vi "WriteIni.vi"(1 "configuration file path":path=path "E:/LabVIEW/福尔达/AppData") -> ()   [LabVIEW 2018]
uses:
  <vilib>/Utility/config.llb/Write Key (Double).vi
  <vilib>/Utility/config.llb/NI_LVConfig.lvlib
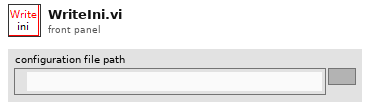
[diagram p1: front panel]
types:
  T1 = typedef "NI_LVConfig.lvlib/Config Data RefNum.ctl" = refnum<k1>
  T2 = cluster{"轮盘预压力":sgl, "泄漏量上限":sgl, "压力上限":sgl, "压力下限":sgl, "风门闭电压上限":sgl, "风门闭电压下限":sgl, "风门开电压上限":sgl, "风门开电压下限":sgl, "LED电流上限":sgl, "LED电流下限":sgl, "气压稳定时间":sgl, "伺服速度":sgl}
  T3 = cluster{"选择":enum16{"Fx", "Fy", "Fz", "Mx", "My", "Mz"}, "系数":sgl, "上限":sgl, "下限":sgl, "Ymax":dbl, "Ymin":dbl, "点数":dbl, "锁系数x":sgl, "锁上限":sgl, "锁下限":sgl, "锁系数+":sgl, "起点":dbl, "终点":dbl, "锁起点":dbl, "锁终点":dbl}
  T4 = cluster{"选择":enum16{"Fx", "Fy", "Fz", "Mx", "My", "Mz"}, "系数":sgl, "上限":sgl, "下限":sgl, "Ymax":dbl, "Ymin":dbl, "点数":dbl, "起点":dbl, "终点":dbl}
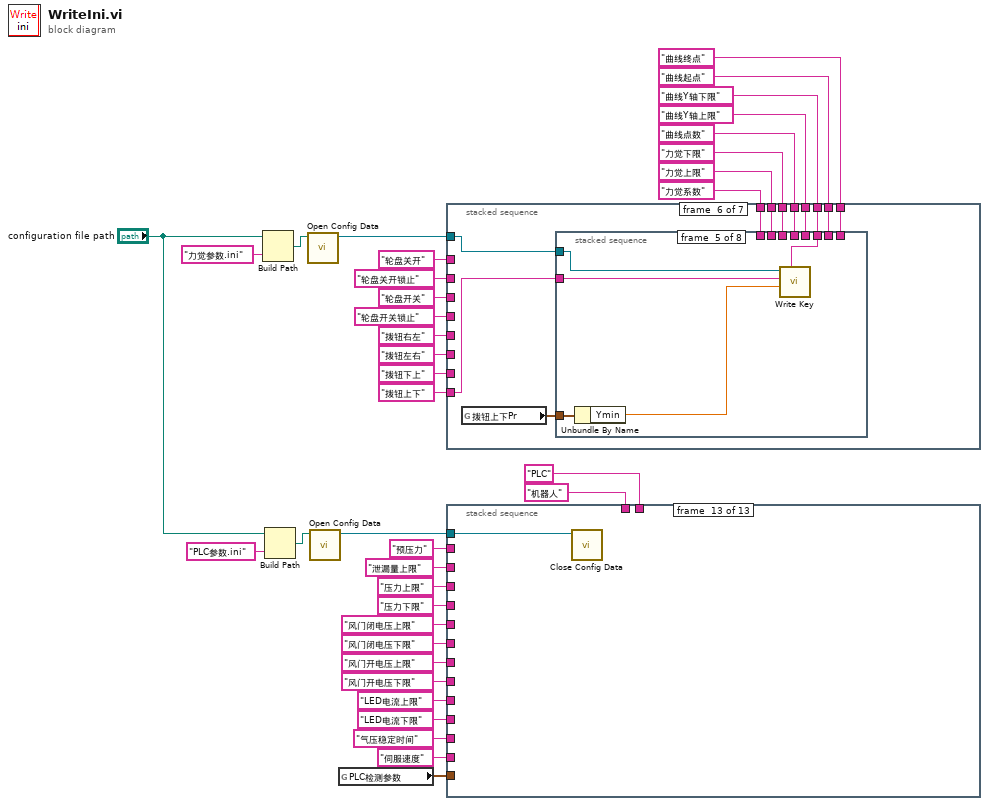
[diagram p0: block diagram]
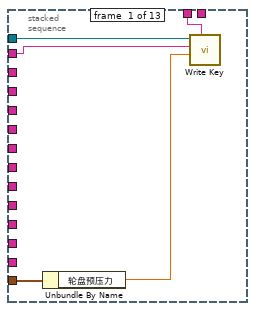
[diagram p2: hidden frame]
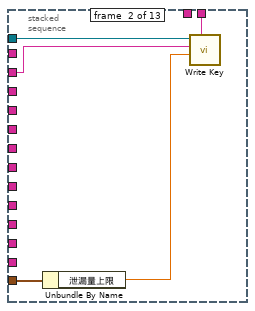
[diagram p3: hidden frame]
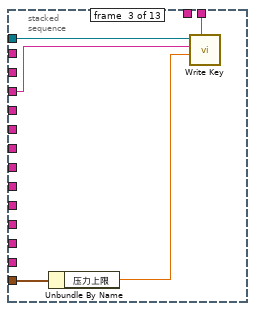
[diagram p4: hidden frame]
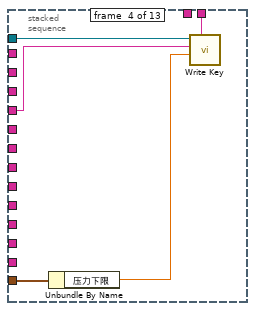
[diagram p5: hidden frame]
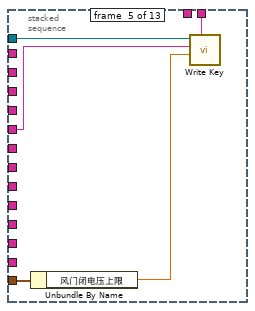
[diagram p6: hidden frame]
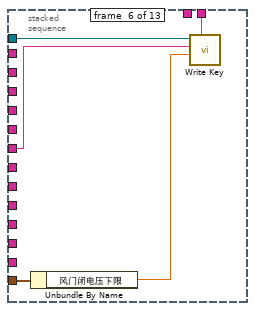
[diagram p7: hidden frame]
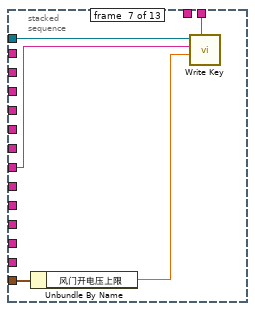
[diagram p8: hidden frame]
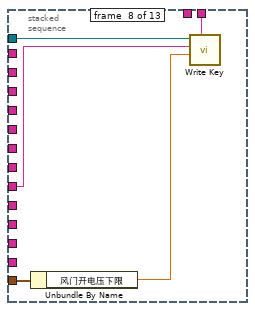
[diagram p9: hidden frame]
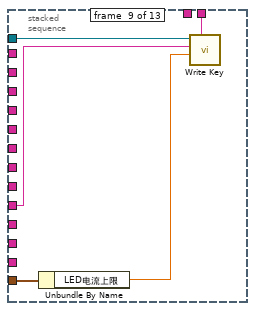
[diagram p10: hidden frame]
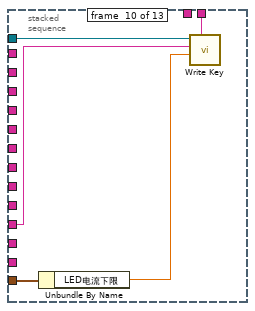
[diagram p11: hidden frame]
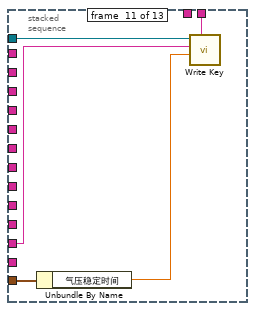
[diagram p12: hidden frame]
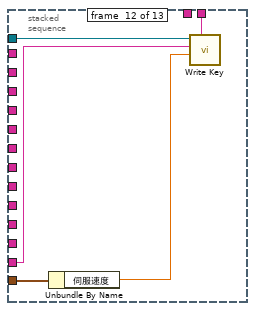
[diagram p13: hidden frame]
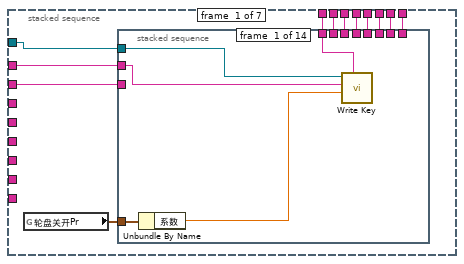
[diagram p14: hidden frame]
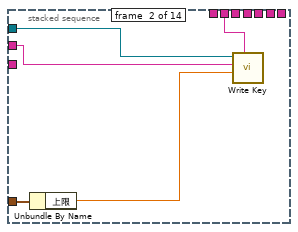
[diagram p15: hidden frame]
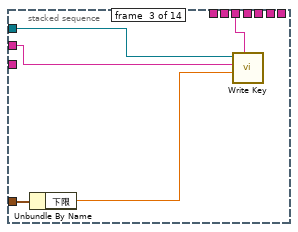
[diagram p16: hidden frame]
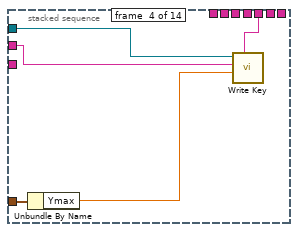
[diagram p17: hidden frame]
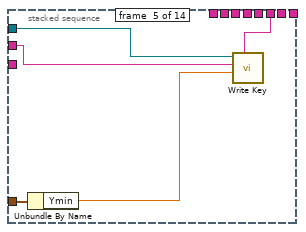
[diagram p18: hidden frame]
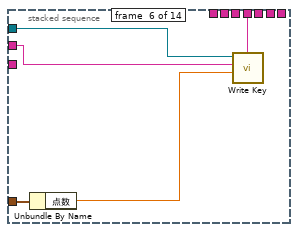
[diagram p19: hidden frame]
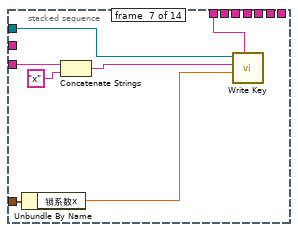
[diagram p20: hidden frame]
diagram:
  n1 = Build Path(base path="configuration file path", name or relative path="力觉参数.ini" ("名称或相对路径")) -> (appended path=w22:path)
  n2 = Build Path(base path="configuration file path", name or relative path="PLC参数.ini" ("名称或相对路径")) -> (appended path=w18:path)
  n3 = call <vilib>:"Open Config Data.vi"("configuration file path"=w22) -> ("refnum"=w20:T1)  [unwired: 8 in, 2 out]
  n4 = call <vilib>:"Open Config Data.vi"("configuration file path"=w18) -> ("refnum"=w17:T1)  [unwired: 8 in, 2 out]
  n5 = global read "全局 1.vi" "PLC检测参数"() -> (w19:T2)
  n6 = stacked-sequence {
    tunnel: w20 -> [w39 w125 w211 w262 w313 w364 w415]
    tunnel: "轮盘关开" -> [w49 _ _ _ _ _ _]
    tunnel: "拨钮上下" -> [_ _ _ _ _ w365 _]
    tunnel: "拨钮下上" -> [_ _ _ _ w314 _ _]
    tunnel: "拨钮左右" -> [_ _ _ w263 _ _ _]
    tunnel: "拨钮右左" -> [_ _ w212 _ _ _ _]
    tunnel: "轮盘开关锁止" -> [_ w126 _ _ _ _ _]
    tunnel: "轮盘开关" -> [_ w127 _ _ _ _ _]
    tunnel: "轮盘关开锁止" -> [w40 _ _ _ _ _ _]
    tunnel: "力觉系数" -> [w48 w135 w220 w271 w322 w373 _]
    tunnel: "力觉上限" -> [w47 w134 w219 w270 w321 w372 _]
    tunnel: "力觉下限" -> [w46 w133 w218 w269 w320 w371 _]
    tunnel: "曲线点数" -> [w45 w132 w217 w268 w319 w370 _]
    tunnel: "曲线Y轴上限" -> [w44 w131 w216 w267 w318 w369 _]
    tunnel: "曲线Y轴下限" -> [w43 w130 w215 w266 w317 w368 _]
    tunnel: "曲线起点" -> [w42 w129 w214 w265 w316 w367 _]
    tunnel: "曲线终点" -> [w41 w128 w213 w264 w315 w366 _]
    frame #0 {
      n7 = global read "全局 1.vi" "轮盘关开Pr"() -> (w50:T3)
      n8 = stacked-sequence {
        tunnel: w49 -> [w52 w57 w62 w67 w72 w77 _ _ _ _ w106 w111 _ _]
        tunnel: w50 -> [w55 w60 w65 w70 w75 w80 w87 w92 w97 w104 w109 w114 w119 w124]
        tunnel: w39 -> [w53 w58 w63 w68 w73 w78 w85 w90 w95 w102 w107 w112 w117 w122]
        tunnel: w48 -> [w51 _ _ _ _ _ w84 _ _ w98 _ _ _ _]
        tunnel: w47 -> [_ w56 _ _ _ _ _ w88 _ _ _ _ _ _]
        tunnel: w46 -> [_ _ w61 _ _ _ _ _ w93 _ _ _ _ _]
        tunnel: w45 -> [_ _ _ _ _ w76 _ _ _ _ _ _ _ _]
        tunnel: w44 -> [_ _ _ w66 _ _ _ _ _ _ _ _ _ _]
        tunnel: w43 -> [_ _ _ _ w71 _ _ _ _ _ _ _ _ _]
        tunnel: w42 -> [_ _ _ _ _ _ _ _ _ _ w105 _ w115 _]
        tunnel: w41 -> [_ _ _ _ _ _ _ _ _ _ _ w110 _ w120]
        tunnel: w40 -> [_ _ _ _ _ _ w83 w89 w94 w101 _ _ w116 w121]
        frame #0 {
          n9 = Unbundle By Name(w55) -> ("系数"=w54:sgl)
          n10 = call-poly <vilib>:"Write Key.vi"("section"=w51, "value"=w54, "key"=w52, "refnum"=w53) -> ()  [unwired: 5 in, 3 out]
        }
        frame #1 {
          n11 = Unbundle By Name(w60) -> ("上限"=w59:sgl)
          n12 = call-poly <vilib>:"Write Key.vi"("section"=w56, "value"=w59, "key"=w57, "refnum"=w58) -> ()  [unwired: 5 in, 3 out]
        }
        frame #2 {
          n13 = Unbundle By Name(w65) -> ("下限"=w64:sgl)
          n14 = call-poly <vilib>:"Write Key.vi"("section"=w61, "value"=w64, "key"=w62, "refnum"=w63) -> ()  [unwired: 5 in, 3 out]
        }
        frame #3 {
          n15 = Unbundle By Name(w70) -> ("Ymax"=w69:dbl)
          n16 = call-poly <vilib>:"Write Key.vi"("section"=w66, "value"=w69, "key"=w67, "refnum"=w68) -> ()  [unwired: 5 in, 3 out]
        }
        frame #4 {
          n17 = Unbundle By Name(w75) -> ("Ymin"=w74:dbl)
          n18 = call-poly <vilib>:"Write Key.vi"("section"=w71, "value"=w74, "key"=w72, "refnum"=w73) -> ()  [unwired: 5 in, 3 out]
        }
        frame #5 {
          n19 = Unbundle By Name(w80) -> ("点数"=w79:dbl)
          n20 = call-poly <vilib>:"Write Key.vi"("section"=w76, "value"=w79, "key"=w77, "refnum"=w78) -> ()  [unwired: 5 in, 3 out]
        }
        frame #6 {
          n21 = Unbundle By Name(w87) -> ("锁系数x"=w86:sgl)
          n22 = Concatenate Strings(w83, "x") -> (w82:string)
          n23 = call-poly <vilib>:"Write Key.vi"("section"=w84, "value"=w86, "key"=w82, "refnum"=w85) -> ()  [unwired: 5 in, 3 out]
        }
        frame #7 {
          n24 = Unbundle By Name(w92) -> ("锁上限"=w91:sgl)
          n25 = call-poly <vilib>:"Write Key.vi"("section"=w88, "value"=w91, "key"=w89, "refnum"=w90) -> ()  [unwired: 5 in, 3 out]
        }
        frame #8 {
          n26 = Unbundle By Name(w97) -> ("锁下限"=w96:sgl)
          n27 = call-poly <vilib>:"Write Key.vi"("section"=w93, "value"=w96, "key"=w94, "refnum"=w95) -> ()  [unwired: 5 in, 3 out]
        }
        frame #9 {
          n28 = Unbundle By Name(w104) -> ("锁系数+"=w103:sgl)
          n29 = Concatenate Strings(w101, "+") -> (w100:string)
          n30 = call-poly <vilib>:"Write Key.vi"("section"=w98, "value"=w103, "key"=w100, "refnum"=w102) -> ()  [unwired: 5 in, 3 out]
        }
        frame #10 {
          n31 = Unbundle By Name(w109) -> ("起点"=w108:dbl)
          n32 = call-poly <vilib>:"Write Key.vi"("section"=w105, "value"=w108, "key"=w106, "refnum"=w107) -> ()  [unwired: 5 in, 3 out]
        }
        frame #11 {
          n33 = Unbundle By Name(w114) -> ("终点"=w113:dbl)
          n34 = call-poly <vilib>:"Write Key.vi"("section"=w110, "value"=w113, "key"=w111, "refnum"=w112) -> ()  [unwired: 5 in, 3 out]
        }
        frame #12 {
          n35 = Unbundle By Name(w119) -> ("锁起点"=w118:dbl)
          n36 = call-poly <vilib>:"Write Key.vi"("section"=w115, "value"=w118, "key"=w116, "refnum"=w117) -> ()  [unwired: 5 in, 3 out]
        }
        frame #13 {
          n37 = Unbundle By Name(w124) -> ("锁终点"=w123:dbl)
          n38 = call-poly <vilib>:"Write Key.vi"("section"=w120, "value"=w123, "key"=w121, "refnum"=w122) -> ()  [unwired: 5 in, 3 out]
        }
      }
    }
    frame #1 {
      n39 = global read "全局 1.vi" "轮盘开关Pr"() -> (w136:T3)
      n40 = stacked-sequence {
        tunnel: w127 -> [w138 w143 w148 w153 w158 w163 _ _ _ _ w192 w197 _ _]
        tunnel: w136 -> [w141 w146 w151 w156 w161 w166 w173 w178 w183 w190 w195 w200 w205 w210]
        tunnel: w125 -> [w139 w144 w149 w154 w159 w164 w171 w176 w181 w188 w193 w198 w203 w208]
        tunnel: w135 -> [w137 _ _ _ _ _ w170 _ _ w184 _ _ _ _]
        tunnel: w134 -> [_ w142 _ _ _ _ _ w174 _ _ _ _ _ _]
        tunnel: w133 -> [_ _ w147 _ _ _ _ _ w179 _ _ _ _ _]
        tunnel: w132 -> [_ _ _ _ _ w162 _ _ _ _ _ _ _ _]
        tunnel: w131 -> [_ _ _ w152 _ _ _ _ _ _ _ _ _ _]
        tunnel: w130 -> [_ _ _ _ w157 _ _ _ _ _ _ _ _ _]
        tunnel: w129 -> [_ _ _ _ _ _ _ _ _ _ w191 _ w201 _]
        tunnel: w128 -> [_ _ _ _ _ _ _ _ _ _ _ w196 _ w206]
        tunnel: w126 -> [_ _ _ _ _ _ w169 w175 w180 w187 _ _ w202 w207]
        frame #0 {
          n41 = Unbundle By Name(w141) -> ("系数"=w140:sgl)
          n42 = call-poly <vilib>:"Write Key.vi"("section"=w137, "value"=w140, "key"=w138, "refnum"=w139) -> ()  [unwired: 5 in, 3 out]
        }
        frame #1 {
          n43 = Unbundle By Name(w146) -> ("上限"=w145:sgl)
          n44 = call-poly <vilib>:"Write Key.vi"("section"=w142, "value"=w145, "key"=w143, "refnum"=w144) -> ()  [unwired: 5 in, 3 out]
        }
        frame #2 {
          n45 = Unbundle By Name(w151) -> ("下限"=w150:sgl)
          n46 = call-poly <vilib>:"Write Key.vi"("section"=w147, "value"=w150, "key"=w148, "refnum"=w149) -> ()  [unwired: 5 in, 3 out]
        }
        frame #3 {
          n47 = Unbundle By Name(w156) -> ("Ymax"=w155:dbl)
          n48 = call-poly <vilib>:"Write Key.vi"("section"=w152, "value"=w155, "key"=w153, "refnum"=w154) -> ()  [unwired: 5 in, 3 out]
        }
        frame #4 {
          n49 = Unbundle By Name(w161) -> ("Ymin"=w160:dbl)
          n50 = call-poly <vilib>:"Write Key.vi"("section"=w157, "value"=w160, "key"=w158, "refnum"=w159) -> ()  [unwired: 5 in, 3 out]
        }
        frame #5 {
          n51 = Unbundle By Name(w166) -> ("点数"=w165:dbl)
          n52 = call-poly <vilib>:"Write Key.vi"("section"=w162, "value"=w165, "key"=w163, "refnum"=w164) -> ()  [unwired: 5 in, 3 out]
        }
        frame #6 {
          n53 = Unbundle By Name(w173) -> ("锁系数x"=w172:sgl)
          n54 = Concatenate Strings(w169, "x") -> (w168:string)
          n55 = call-poly <vilib>:"Write Key.vi"("section"=w170, "value"=w172, "key"=w168, "refnum"=w171) -> ()  [unwired: 5 in, 3 out]
        }
        frame #7 {
          n56 = Unbundle By Name(w178) -> ("锁上限"=w177:sgl)
          n57 = call-poly <vilib>:"Write Key.vi"("section"=w174, "value"=w177, "key"=w175, "refnum"=w176) -> ()  [unwired: 5 in, 3 out]
        }
        frame #8 {
          n58 = Unbundle By Name(w183) -> ("锁下限"=w182:sgl)
          n59 = call-poly <vilib>:"Write Key.vi"("section"=w179, "value"=w182, "key"=w180, "refnum"=w181) -> ()  [unwired: 5 in, 3 out]
        }
        frame #9 {
          n60 = Unbundle By Name(w190) -> ("锁系数+"=w189:sgl)
          n61 = Concatenate Strings(w187, "+") -> (w186:string)
          n62 = call-poly <vilib>:"Write Key.vi"("section"=w184, "value"=w189, "key"=w186, "refnum"=w188) -> ()  [unwired: 5 in, 3 out]
        }
        frame #10 {
          n63 = Unbundle By Name(w195) -> ("起点"=w194:dbl)
          n64 = call-poly <vilib>:"Write Key.vi"("section"=w191, "value"=w194, "key"=w192, "refnum"=w193) -> ()  [unwired: 5 in, 3 out]
        }
        frame #11 {
          n65 = Unbundle By Name(w200) -> ("终点"=w199:dbl)
          n66 = call-poly <vilib>:"Write Key.vi"("section"=w196, "value"=w199, "key"=w197, "refnum"=w198) -> ()  [unwired: 5 in, 3 out]
        }
        frame #12 {
          n67 = Unbundle By Name(w205) -> ("锁起点"=w204:dbl)
          n68 = call-poly <vilib>:"Write Key.vi"("section"=w201, "value"=w204, "key"=w202, "refnum"=w203) -> ()  [unwired: 5 in, 3 out]
        }
        frame #13 {
          n69 = Unbundle By Name(w210) -> ("锁终点"=w209:dbl)
          n70 = call-poly <vilib>:"Write Key.vi"("section"=w206, "value"=w209, "key"=w207, "refnum"=w208) -> ()  [unwired: 5 in, 3 out]
        }
      }
    }
    frame #2 {
      n71 = global read "全局 1.vi" "拨钮右左Pr"() -> (w221:T4)
      n72 = stacked-sequence {
        tunnel: w212 -> [w223 w228 w233 w238 w243 w248 w253 w258]
        tunnel: w221 -> [w226 w231 w236 w241 w246 w251 w256 w261]
        tunnel: w211 -> [w224 w229 w234 w239 w244 w249 w254 w259]
        tunnel: w220 -> [w222 _ _ _ _ _ _ _]
        tunnel: w219 -> [_ w227 _ _ _ _ _ _]
        tunnel: w218 -> [_ _ w232 _ _ _ _ _]
        tunnel: w217 -> [_ _ _ _ _ w247 _ _]
        tunnel: w216 -> [_ _ _ w237 _ _ _ _]
        tunnel: w215 -> [_ _ _ _ w242 _ _ _]
        tunnel: w214 -> [_ _ _ _ _ _ w252 _]
        tunnel: w213 -> [_ _ _ _ _ _ _ w257]
        frame #0 {
          n73 = Unbundle By Name(w226) -> ("系数"=w225:sgl)
          n74 = call-poly <vilib>:"Write Key.vi"("section"=w222, "value"=w225, "key"=w223, "refnum"=w224) -> ()  [unwired: 5 in, 3 out]
        }
        frame #1 {
          n75 = Unbundle By Name(w231) -> ("上限"=w230:sgl)
          n76 = call-poly <vilib>:"Write Key.vi"("section"=w227, "value"=w230, "key"=w228, "refnum"=w229) -> ()  [unwired: 5 in, 3 out]
        }
        frame #2 {
          n77 = Unbundle By Name(w236) -> ("下限"=w235:sgl)
          n78 = call-poly <vilib>:"Write Key.vi"("section"=w232, "value"=w235, "key"=w233, "refnum"=w234) -> ()  [unwired: 5 in, 3 out]
        }
        frame #3 {
          n79 = Unbundle By Name(w241) -> ("Ymax"=w240:dbl)
          n80 = call-poly <vilib>:"Write Key.vi"("section"=w237, "value"=w240, "key"=w238, "refnum"=w239) -> ()  [unwired: 5 in, 3 out]
        }
        frame #4 {
          n81 = Unbundle By Name(w246) -> ("Ymin"=w245:dbl)
          n82 = call-poly <vilib>:"Write Key.vi"("section"=w242, "value"=w245, "key"=w243, "refnum"=w244) -> ()  [unwired: 5 in, 3 out]
        }
        frame #5 {
          n83 = Unbundle By Name(w251) -> ("点数"=w250:dbl)
          n84 = call-poly <vilib>:"Write Key.vi"("section"=w247, "value"=w250, "key"=w248, "refnum"=w249) -> ()  [unwired: 5 in, 3 out]
        }
        frame #6 {
          n85 = Unbundle By Name(w256) -> ("起点"=w255:dbl)
          n86 = call-poly <vilib>:"Write Key.vi"("section"=w252, "value"=w255, "key"=w253, "refnum"=w254) -> ()  [unwired: 5 in, 3 out]
        }
        frame #7 {
          n87 = Unbundle By Name(w261) -> ("终点"=w260:dbl)
          n88 = call-poly <vilib>:"Write Key.vi"("section"=w257, "value"=w260, "key"=w258, "refnum"=w259) -> ()  [unwired: 5 in, 3 out]
        }
      }
    }
    frame #3 {
      n89 = global read "全局 1.vi" "拨钮左右Pr"() -> (w272:T4)
      n90 = stacked-sequence {
        tunnel: w263 -> [w274 w279 w284 w289 w294 w299 w304 w309]
        tunnel: w272 -> [w277 w282 w287 w292 w297 w302 w307 w312]
        tunnel: w262 -> [w275 w280 w285 w290 w295 w300 w305 w310]
        tunnel: w271 -> [w273 _ _ _ _ _ _ _]
        tunnel: w270 -> [_ w278 _ _ _ _ _ _]
        tunnel: w269 -> [_ _ w283 _ _ _ _ _]
        tunnel: w268 -> [_ _ _ _ _ w298 _ _]
        tunnel: w267 -> [_ _ _ w288 _ _ _ _]
        tunnel: w266 -> [_ _ _ _ w293 _ _ _]
        tunnel: w265 -> [_ _ _ _ _ _ w303 _]
        tunnel: w264 -> [_ _ _ _ _ _ _ w308]
        frame #0 {
          n91 = Unbundle By Name(w277) -> ("系数"=w276:sgl)
          n92 = call-poly <vilib>:"Write Key.vi"("section"=w273, "value"=w276, "key"=w274, "refnum"=w275) -> ()  [unwired: 5 in, 3 out]
        }
        frame #1 {
          n93 = Unbundle By Name(w282) -> ("上限"=w281:sgl)
          n94 = call-poly <vilib>:"Write Key.vi"("section"=w278, "value"=w281, "key"=w279, "refnum"=w280) -> ()  [unwired: 5 in, 3 out]
        }
        frame #2 {
          n95 = Unbundle By Name(w287) -> ("下限"=w286:sgl)
          n96 = call-poly <vilib>:"Write Key.vi"("section"=w283, "value"=w286, "key"=w284, "refnum"=w285) -> ()  [unwired: 5 in, 3 out]
        }
        frame #3 {
          n97 = Unbundle By Name(w292) -> ("Ymax"=w291:dbl)
          n98 = call-poly <vilib>:"Write Key.vi"("section"=w288, "value"=w291, "key"=w289, "refnum"=w290) -> ()  [unwired: 5 in, 3 out]
        }
        frame #4 {
          n99 = Unbundle By Name(w297) -> ("Ymin"=w296:dbl)
          n100 = call-poly <vilib>:"Write Key.vi"("section"=w293, "value"=w296, "key"=w294, "refnum"=w295) -> ()  [unwired: 5 in, 3 out]
        }
        frame #5 {
          n101 = Unbundle By Name(w302) -> ("点数"=w301:dbl)
          n102 = call-poly <vilib>:"Write Key.vi"("section"=w298, "value"=w301, "key"=w299, "refnum"=w300) -> ()  [unwired: 5 in, 3 out]
        }
        frame #6 {
          n103 = Unbundle By Name(w307) -> ("起点"=w306:dbl)
          n104 = call-poly <vilib>:"Write Key.vi"("section"=w303, "value"=w306, "key"=w304, "refnum"=w305) -> ()  [unwired: 5 in, 3 out]
        }
        frame #7 {
          n105 = Unbundle By Name(w312) -> ("终点"=w311:dbl)
          n106 = call-poly <vilib>:"Write Key.vi"("section"=w308, "value"=w311, "key"=w309, "refnum"=w310) -> ()  [unwired: 5 in, 3 out]
        }
      }
    }
    frame #4 {
      n107 = global read "全局 1.vi" "拨钮下上Pr"() -> (w323:T4)
      n108 = stacked-sequence {
        tunnel: w314 -> [w325 w330 w335 w340 w345 w350 w355 w360]
        tunnel: w323 -> [w328 w333 w338 w343 w348 w353 w358 w363]
        tunnel: w313 -> [w326 w331 w336 w341 w346 w351 w356 w361]
        tunnel: w322 -> [w324 _ _ _ _ _ _ _]
        tunnel: w321 -> [_ w329 _ _ _ _ _ _]
        tunnel: w320 -> [_ _ w334 _ _ _ _ _]
        tunnel: w319 -> [_ _ _ _ _ w349 _ _]
        tunnel: w318 -> [_ _ _ w339 _ _ _ _]
        tunnel: w317 -> [_ _ _ _ w344 _ _ _]
        tunnel: w316 -> [_ _ _ _ _ _ w354 _]
        tunnel: w315 -> [_ _ _ _ _ _ _ w359]
        frame #0 {
          n109 = Unbundle By Name(w328) -> ("系数"=w327:sgl)
          n110 = call-poly <vilib>:"Write Key.vi"("section"=w324, "value"=w327, "key"=w325, "refnum"=w326) -> ()  [unwired: 5 in, 3 out]
        }
        frame #1 {
          n111 = Unbundle By Name(w333) -> ("上限"=w332:sgl)
          n112 = call-poly <vilib>:"Write Key.vi"("section"=w329, "value"=w332, "key"=w330, "refnum"=w331) -> ()  [unwired: 5 in, 3 out]
        }
        frame #2 {
          n113 = Unbundle By Name(w338) -> ("下限"=w337:sgl)
          n114 = call-poly <vilib>:"Write Key.vi"("section"=w334, "value"=w337, "key"=w335, "refnum"=w336) -> ()  [unwired: 5 in, 3 out]
        }
        frame #3 {
          n115 = Unbundle By Name(w343) -> ("Ymax"=w342:dbl)
          n116 = call-poly <vilib>:"Write Key.vi"("section"=w339, "value"=w342, "key"=w340, "refnum"=w341) -> ()  [unwired: 5 in, 3 out]
        }
        frame #4 {
          n117 = Unbundle By Name(w348) -> ("Ymin"=w347:dbl)
          n118 = call-poly <vilib>:"Write Key.vi"("section"=w344, "value"=w347, "key"=w345, "refnum"=w346) -> ()  [unwired: 5 in, 3 out]
        }
        frame #5 {
          n119 = Unbundle By Name(w353) -> ("点数"=w352:dbl)
          n120 = call-poly <vilib>:"Write Key.vi"("section"=w349, "value"=w352, "key"=w350, "refnum"=w351) -> ()  [unwired: 5 in, 3 out]
        }
        frame #6 {
          n121 = Unbundle By Name(w358) -> ("起点"=w357:dbl)
          n122 = call-poly <vilib>:"Write Key.vi"("section"=w354, "value"=w357, "key"=w355, "refnum"=w356) -> ()  [unwired: 5 in, 3 out]
        }
        frame #7 {
          n123 = Unbundle By Name(w363) -> ("终点"=w362:dbl)
          n124 = call-poly <vilib>:"Write Key.vi"("section"=w359, "value"=w362, "key"=w360, "refnum"=w361) -> ()  [unwired: 5 in, 3 out]
        }
      }
    }
    frame #5 {
      n125 = global read "全局 1.vi" "拨钮上下Pr"() -> (w374:T4)
      n126 = stacked-sequence {
        tunnel: w365 -> [w376 w381 w386 w391 w396 w401 w406 w411]
        tunnel: w374 -> [w379 w384 w389 w394 w399 w404 w409 w414]
        tunnel: w364 -> [w377 w382 w387 w392 w397 w402 w407 w412]
        tunnel: w373 -> [w375 _ _ _ _ _ _ _]
        tunnel: w372 -> [_ w380 _ _ _ _ _ _]
        tunnel: w371 -> [_ _ w385 _ _ _ _ _]
        tunnel: w370 -> [_ _ _ _ _ w400 _ _]
        tunnel: w369 -> [_ _ _ w390 _ _ _ _]
        tunnel: w368 -> [_ _ _ _ w395 _ _ _]
        tunnel: w367 -> [_ _ _ _ _ _ w405 _]
        tunnel: w366 -> [_ _ _ _ _ _ _ w410]
        frame #0 {
          n127 = Unbundle By Name(w379) -> ("系数"=w378:sgl)
          n128 = call-poly <vilib>:"Write Key.vi"("section"=w375, "value"=w378, "key"=w376, "refnum"=w377) -> ()  [unwired: 5 in, 3 out]
        }
        frame #1 {
          n129 = Unbundle By Name(w384) -> ("上限"=w383:sgl)
          n130 = call-poly <vilib>:"Write Key.vi"("section"=w380, "value"=w383, "key"=w381, "refnum"=w382) -> ()  [unwired: 5 in, 3 out]
        }
        frame #2 {
          n131 = Unbundle By Name(w389) -> ("下限"=w388:sgl)
          n132 = call-poly <vilib>:"Write Key.vi"("section"=w385, "value"=w388, "key"=w386, "refnum"=w387) -> ()  [unwired: 5 in, 3 out]
        }
        frame #3 {
          n133 = Unbundle By Name(w394) -> ("Ymax"=w393:dbl)
          n134 = call-poly <vilib>:"Write Key.vi"("section"=w390, "value"=w393, "key"=w391, "refnum"=w392) -> ()  [unwired: 5 in, 3 out]
        }
        frame #4 {
          n135 = Unbundle By Name(w399) -> ("Ymin"=w398:dbl)
          n136 = call-poly <vilib>:"Write Key.vi"("section"=w395, "value"=w398, "key"=w396, "refnum"=w397) -> ()  [unwired: 5 in, 3 out]
        }
        frame #5 {
          n137 = Unbundle By Name(w404) -> ("点数"=w403:dbl)
          n138 = call-poly <vilib>:"Write Key.vi"("section"=w400, "value"=w403, "key"=w401, "refnum"=w402) -> ()  [unwired: 5 in, 3 out]
        }
        frame #6 {
          n139 = Unbundle By Name(w409) -> ("起点"=w408:dbl)
          n140 = call-poly <vilib>:"Write Key.vi"("section"=w405, "value"=w408, "key"=w406, "refnum"=w407) -> ()  [unwired: 5 in, 3 out]
        }
        frame #7 {
          n141 = Unbundle By Name(w414) -> ("终点"=w413:dbl)
          n142 = call-poly <vilib>:"Write Key.vi"("section"=w410, "value"=w413, "key"=w411, "refnum"=w412) -> ()  [unwired: 5 in, 3 out]
        }
      }
    }
    frame #6 {
      n143 = call <vilib>:"Close Config Data.vi"("refnum"=w415) -> ()  [unwired: 9 in, 2 out]
    }
  }
  n144 = stacked-sequence {
    tunnel: w19 -> [w420 w425 w430 w435 w440 w445 w450 w455 w460 w465 w470 w475 _]
    tunnel: w17 -> [w418 w423 w428 w433 w438 w443 w448 w453 w458 w463 w468 w473 w476]
    tunnel: "预压力" -> [w416 _ _ _ _ _ _ _ _ _ _ _ _]
    tunnel: "泄漏量上限" -> [_ w422 _ _ _ _ _ _ _ _ _ _ _]
    tunnel: "压力上限" -> [_ _ w426 _ _ _ _ _ _ _ _ _ _]
    tunnel: "压力下限" -> [_ _ _ w431 _ _ _ _ _ _ _ _ _]
    tunnel: "风门闭电压上限" -> [_ _ _ _ w436 _ _ _ _ _ _ _ _]
    tunnel: "风门闭电压下限" -> [_ _ _ _ _ w441 _ _ _ _ _ _ _]
    tunnel: "风门开电压上限" -> [_ _ _ _ _ _ w446 _ _ _ _ _ _]
    tunnel: "风门开电压下限" -> [_ _ _ _ _ _ _ w451 _ _ _ _ _]
    tunnel: "LED电流上限" -> [_ _ _ _ _ _ _ _ w456 _ _ _ _]
    tunnel: "LED电流下限" -> [_ _ _ _ _ _ _ _ _ w461 _ _ _]
    tunnel: "气压稳定时间" -> [_ _ _ _ _ _ _ _ _ _ w466 _ _]
    tunnel: "伺服速度" -> [_ _ _ _ _ _ _ _ _ _ _ w471 _]
    tunnel: "机器人" -> [w417 _ _ _ _ _ _ _ _ _ _ _ _]
    tunnel: "PLC" -> [_ w421 w427 w432 w437 w442 w447 w452 w457 w462 w467 w472 _]
    frame #0 {
      n145 = Unbundle By Name(w420) -> ("轮盘预压力"=w419:sgl)
      n146 = call-poly <vilib>:"Write Key.vi"("section"=w417, "value"=w419, "key"=w416, "refnum"=w418) -> ()  [unwired: 5 in, 3 out]
    }
    frame #1 {
      n147 = Unbundle By Name(w425) -> ("泄漏量上限"=w424:sgl)
      n148 = call-poly <vilib>:"Write Key.vi"("section"=w421, "value"=w424, "key"=w422, "refnum"=w423) -> ()  [unwired: 5 in, 3 out]
    }
    frame #2 {
      n149 = Unbundle By Name(w430) -> ("压力上限"=w429:sgl)
      n150 = call-poly <vilib>:"Write Key.vi"("section"=w427, "value"=w429, "key"=w426, "refnum"=w428) -> ()  [unwired: 5 in, 3 out]
    }
    frame #3 {
      n151 = Unbundle By Name(w435) -> ("压力下限"=w434:sgl)
      n152 = call-poly <vilib>:"Write Key.vi"("section"=w432, "value"=w434, "key"=w431, "refnum"=w433) -> ()  [unwired: 5 in, 3 out]
    }
    frame #4 {
      n153 = Unbundle By Name(w440) -> ("风门闭电压上限"=w439:sgl)
      n154 = call-poly <vilib>:"Write Key.vi"("section"=w437, "value"=w439, "key"=w436, "refnum"=w438) -> ()  [unwired: 5 in, 3 out]
    }
    frame #5 {
      n155 = Unbundle By Name(w445) -> ("风门闭电压下限"=w444:sgl)
      n156 = call-poly <vilib>:"Write Key.vi"("section"=w442, "value"=w444, "key"=w441, "refnum"=w443) -> ()  [unwired: 5 in, 3 out]
    }
    frame #6 {
      n157 = Unbundle By Name(w450) -> ("风门开电压上限"=w449:sgl)
      n158 = call-poly <vilib>:"Write Key.vi"("section"=w447, "value"=w449, "key"=w446, "refnum"=w448) -> ()  [unwired: 5 in, 3 out]
    }
    frame #7 {
      n159 = Unbundle By Name(w455) -> ("风门开电压下限"=w454:sgl)
      n160 = call-poly <vilib>:"Write Key.vi"("section"=w452, "value"=w454, "key"=w451, "refnum"=w453) -> ()  [unwired: 5 in, 3 out]
    }
    frame #8 {
      n161 = Unbundle By Name(w460) -> ("LED电流上限"=w459:sgl)
      n162 = call-poly <vilib>:"Write Key.vi"("section"=w457, "value"=w459, "key"=w456, "refnum"=w458) -> ()  [unwired: 5 in, 3 out]
    }
    frame #9 {
      n163 = Unbundle By Name(w465) -> ("LED电流下限"=w464:sgl)
      n164 = call-poly <vilib>:"Write Key.vi"("section"=w462, "value"=w464, "key"=w461, "refnum"=w463) -> ()  [unwired: 5 in, 3 out]
    }
    frame #10 {
      n165 = Unbundle By Name(w470) -> ("气压稳定时间"=w469:sgl)
      n166 = call-poly <vilib>:"Write Key.vi"("section"=w467, "value"=w469, "key"=w466, "refnum"=w468) -> ()  [unwired: 5 in, 3 out]
    }
    frame #11 {
      n167 = Unbundle By Name(w475) -> ("伺服速度"=w474:sgl)
      n168 = call-poly <vilib>:"Write Key.vi"("section"=w472, "value"=w474, "key"=w471, "refnum"=w473) -> ()  [unwired: 5 in, 3 out]
    }
    frame #12 {
      n169 = call <vilib>:"Close Config Data.vi"("refnum"=w476) -> ()  [unwired: 9 in, 2 out]
    }
  }
